vi "Open.vi"(8 "error in (no error)":errorcluster, 10 "Interface_type":T1="DALI", 11 "Toolbox in":refnum<class "Toolbox.lvclass">) -> (0 "error out":errorcluster, 3 "Toolbox out":refnum<class "Toolbox.lvclass">)   [LabVIEW 2014, in "Driver_interaction.lvlib" / "Toolbox.lvclass"]
uses:
  Toolbox.lvclass
  _Driver_interaction/Controls/Interface_type.ctl
  Vendor/lib 2p0/types/interface_type.ctl
  Controls/Toolbox_session.ctl
  <vilib>/httpClient/ClientHandle.ctl
  _Driver_interaction/_Driver_interaction.lvclass/_Driver_interaction.ctl
  Toolbox.lvclass/Toolbox.ctl
  _Driver_interaction/_Driver_interaction.lvclass
  Deploy/Utilities/Miscelanous.lvlibp
  Vendor/lib 2p0/FTS 2p0.lvlib
  <vilib>/httpClient/LabVIEWHTTPClient.lvlib
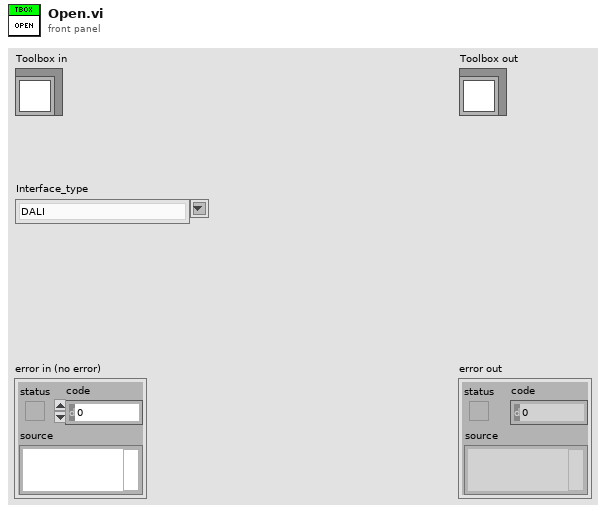
[diagram p1: front panel]
types:
  T1 = typedef "Driver_interaction.lvlib/_Driver_interaction.lvclass/Interface_type.ctl" = string
  T2 = typedef "Driver_interaction.lvlib/Toolbox.lvclass/Toolbox_session.ctl" = cluster{"client handle":T3, "URL out":string, "universe_id":i32, "devices_id":i32[]}
  T3 = typedef "LabVIEWHTTPClient.lvlib/ClientHandle.ctl" = refnum<k1>
  T4 = typedef "FTS 2p0.lvlib/interface_type.ctl" = string
  T5 = cluster{"result":cluster{"interface_type":T4, "parent_device_id":string, "universe_id":i32, "universe_name":string}[]}
  T6 = cluster{"interface_type":T4, "parent_device_id":string, "universe_id":i32, "universe_name":string}[]
  T7 = cluster{"interface_type":T4, "parent_device_id":string, "universe_id":i32, "universe_name":string}
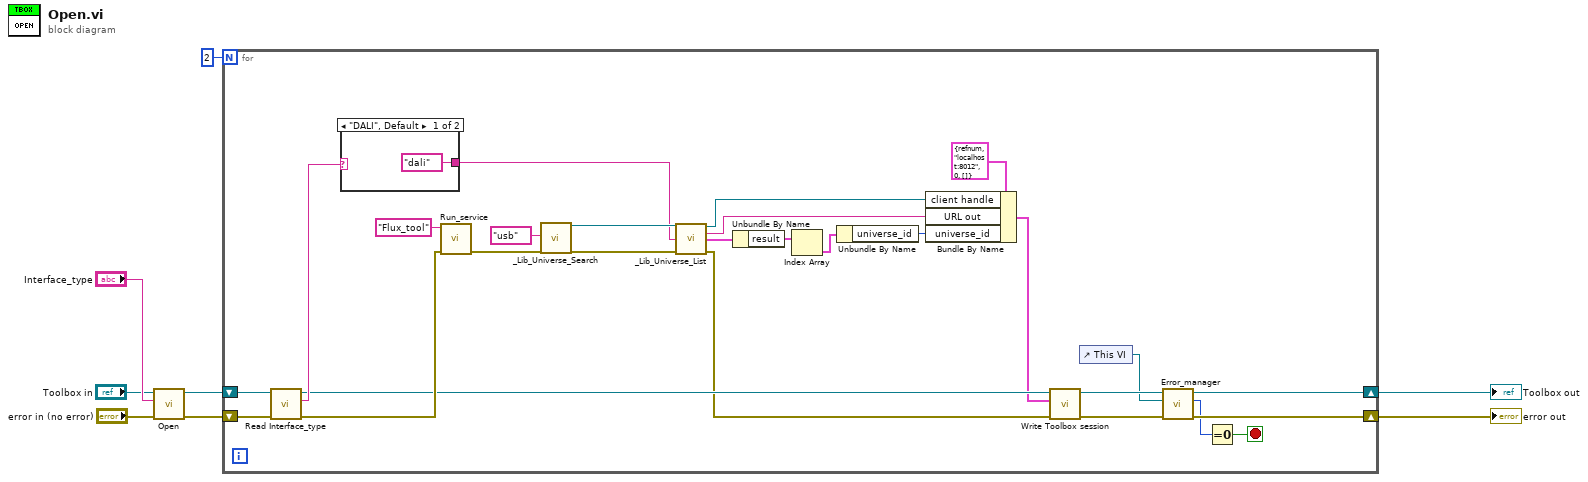
[diagram p0: block diagram]
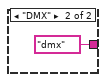
[diagram p2: hidden frame]
diagram:
  n1 = call-parent "Open.vi"("error in (no error)"="error in (no error)", "Interface_type"="Interface_type", "_Driver_interaction in"="Toolbox in") -> ("error out"=w5:errorcluster, "_Driver_interaction out"=w4:refnum<class "Toolbox.lvclass">)  [unwired: 7 in]
  n2 = for {
    N: 2 -> [_]
    shift-right: [w12] -> w2
    shift-left: w5 -> [w32]
    shift-right: [w13] -> w3
    shift-left: w4 -> [w31]
    stop <- w10 stop-if-true
    n3 = call "Read Interface_type.vi"("error in (no error)"=w32, "_Driver_interaction in"=w31) -> ("error out"=w22:errorcluster, "Interface_type"=w28:T1, "_Driver_interaction out"=w21:refnum<class "Toolbox.lvclass">)  [unwired: 7 in]
    n4 = case shown="\"DALI\", Default" w28 {
      tunnel: [T4 "dali" ("params.interface_type") T4 "dmx" ("params.interface_type")] -> w18
      frame "DALI", Default {
      }
      frame "DMX" {
      }
    }
    n5 = call "Run_service.vi"("error in (no error)"=w22, "Service"="Flux_tool") -> ("error out"=w34:errorcluster)  [unwired: 8 in, 1 out]
    n6 = call "_Lib_Universe_Search.vi"("params.interface_type"=T4 "usb", "error in (no error)"=w34) -> ("client handle out"=w30:T3, "error out"=w33:errorcluster)  [unwired: 13 in, 3 out]
    n7 = call "_Lib_Universe_List.vi"("client handle"=w30, "params.interface_type"=w18, "error in (no error)"=w33) -> ("client handle out"=w26:T3, "URL out"=w25:string, "universe"=w17:T5, "error out"=w20:errorcluster)  [unwired: 9 in]
    n8 = Unbundle By Name(w17) -> ("result"=w24:T6)
    n9 = Index Array(array=w24) -> (element=w16:T7)  [unwired: 1 in]
    n10 = Unbundle By Name(w16) -> ("universe_id"=w23:i32)
    n11 = Bundle By Name(cluster=T2 {"client handle"=refnum, "URL out"="localhost:8012", "universe_id"=0, "devices_id"=[]} ("Toolbox session"), "client handle"=w26, "URL out"=w25, "universe_id"=w23) -> (w19:T2)
    n12 = call "Write Toolbox session.vi"("error in (no error)"=w20, "Toolbox session"=w19, "Toolbox in"=w21) -> ("error out"=w15:errorcluster, "Toolbox out"=w14:refnum<class "Toolbox.lvclass">)  [unwired: 7 in]
    n13 = control-ref of="This VI"() -> (w11:refnum<vi>)
    n14 = call-dynamic "Error_manager.vi"("error in (no error)"=w15, "Caller VI"=w11, "Toolbox in"=w14) -> ("error out"=w12:errorcluster, "code"=w9:i32, "Toolbox out"=w13:refnum<class "Toolbox.lvclass">)  [unwired: 4 in, 2 out]
    n15 = Equal To 0?(x=w9) -> (x = 0?=w10:bool)
  }
  "error out" <- w2
  "Toolbox out" <- w3
